vi "Grid_Init_v2.vi"(7 "resume":T1, 8 "Error in":errorcluster, 10 "Settings":T2={"Drift Correction Settings"={"Drift Correction every"=80, "Drift correction Pixels"=256, "Channel index (0-23)"=0, "MaxImagesBack"=2, "Threshold"=2, "Increment"=8, "max applied Drift Correction"=20, "Correct Drift"=TRUE, "Correlate"=0, "Correct z drift"=FALSE, "zdrift \nDuration (s)"=0.0}, "Spectroscopy Setting"={"Imaging Current"=1e-11, "ref Current"=7e-11, "tip Speed (m/s)"=2e-09, "Imaging Bias"=0.02, "ref Bias"=-0.1, "preSTS delay [ms]"=500, "STS z offset"=2e-10, "during Spec Bias (V)"=-0.1, "trigger1 < Hz"=0.0, "trigger 2 >Hz"=0.0, "autoStop"=FALSE, "Spectroscopy"=0, "PLL ON/OFF"=TRUE, "readjust setpoint every "=1, "z Reference"=FALSE, "Lock In"=TRUE}, "Misc"={"File name"="symmetric_node_zOff=200p", "Email when finished"="cornelius.krull@monash.edu,Dhaneesh.Gopalakrishnan@monash.edu,marina.castelli@monash.edu"}, "Grid Settings"={"type"=1, "type order"=1, "X pixel"=0, "Y pixel"=0, "Grid_Parms"={"center X (m)"=0.0, "center Y (m)"=0.0, "width (m)"=0.0, "height (m)"=0.0, "angle (deg)"=0.0}}} {"Grid Settings"."type order" items=["Line", "Grid"]; "Grid Settings"."type" items=["Line", "Grid"]; "Spectroscopy Setting"."Spectroscopy" items=["Bias", "zSpec"]; "Spectroscopy Setting"."trigger 2 >Hz" format="%#_6p"; "Spectroscopy Setting"."trigger1 < Hz" format="%#_6p"; "Spectroscopy Setting"."during Spec Bias (V)" format="%#_5p"; "Spectroscopy Setting"."STS z offset" format="%#_6p"; "Spectroscopy Setting"."ref Bias" format="%#_6p"; "Spectroscopy Setting"."Imaging Bias" format="%#_6p"; "Spectroscopy Setting"."tip Speed (m/s)" format="%.2p"; "Spectroscopy Setting"."ref Current" format="%#_6p"; "Spectroscopy Setting"."Imaging Current" format="%#_6p"; "Drift Correction Settings"."Correlate" items=["first Frame", "successive Frames"]; "Drift Correction Settings"."max applied Drift Correction" min=1 max=100 step=1 format="%.0p"; "Drift Correction Settings"."Threshold" min=1 step=1; "Drift Correction Settings"."Channel index (0-23)" items=["Current"=0, "Z (m)"=14]}, 11 "Application reference":refnum<vi>) -> (0 "error out":errorcluster, 1 "FileRefs":T3, 2 "Settings out":T2={"Drift Correction Settings"={"Drift Correction every"=80, "Drift correction Pixels"=256, "Channel index (0-23)"=0, "MaxImagesBack"=2, "Threshold"=2, "Increment"=8, "max applied Drift Correction"=20, "Correct Drift"=TRUE, "Correlate"=0, "Correct z drift"=FALSE, "zdrift \nDuration (s)"=0.0}, "Spectroscopy Setting"={"Imaging Current"=1e-11, "ref Current"=7e-11, "tip Speed (m/s)"=2e-09, "Imaging Bias"=0.02, "ref Bias"=-0.1, "preSTS delay [ms]"=500, "STS z offset"=2e-10, "during Spec Bias (V)"=-0.1, "trigger1 < Hz"=0.0, "trigger 2 >Hz"=0.0, "autoStop"=FALSE, "Spectroscopy"=0, "PLL ON/OFF"=TRUE, "readjust setpoint every "=1, "z Reference"=FALSE, "Lock In"=TRUE}, "Misc"={"File name"="symmetric_node_zOff=200p", "Email when finished"="cornelius.krull@monash.edu,Dhaneesh.Gopalakrishnan@monash.edu,marina.castelli@monash.edu"}, "Grid Settings"={"type"=1, "type order"=1, "X pixel"=0, "Y pixel"=0, "Grid_Parms"={"center X (m)"=0.0, "center Y (m)"=0.0, "width (m)"=0.0, "height (m)"=0.0, "angle (deg)"=0.0}}} caption="Settings" {"Grid Settings"."type order" items=["Line", "Grid"]; "Grid Settings"."type" items=["Line", "Grid"]; "Spectroscopy Setting"."Spectroscopy" items=["Bias", "zSpec"]; "Spectroscopy Setting"."trigger 2 >Hz" format="%#_6p"; "Spectroscopy Setting"."trigger1 < Hz" format="%#_6p"; "Spectroscopy Setting"."during Spec Bias (V)" format="%#_5p"; "Spectroscopy Setting"."STS z offset" format="%#_6p"; "Spectroscopy Setting"."ref Bias" format="%#_6p"; "Spectroscopy Setting"."Imaging Bias" format="%#_6p"; "Spectroscopy Setting"."tip Speed (m/s)" format="%.2p"; "Spectroscopy Setting"."ref Current" format="%#_6p"; "Spectroscopy Setting"."Imaging Current" format="%#_6p"; "Drift Correction Settings"."Correlate" items=["first Frame", "successive Frames"]; "Drift Correction Settings"."max applied Drift Correction" min=1 max=100 step=1 format="%.0p"; "Drift Correction Settings"."Threshold" min=1 step=1; "Drift Correction Settings"."Channel index (0-23)" items=["Current"=0, "Z (m)"=14]}, 3 "Application ref out":refnum<vi>, 5 "DC images":dbl[][][](array[numeric]))   [LabVIEW 2014]
uses:
  <userlib>/Nanonis Prog Interface V5/Nanonis Prog Interface.lvlib
panel:
  # "RUN smart tilt before starting the GRID\nImg Angle = 0  CHECK CUTOFF\nmove tip to reference point for tip height"
  # "z Spectroscopy"
  # "GRID points"
  # "Increase this if no Drift was detected for \na certain number of images"
  # "% of image size"
  # "RUN smart tilt before starting the GRID\nImg Angle = 0  CHECK CUTOFF\nmove tip to reference point for tip height"
  # "z Spectroscopy"
  # "GRID points"
  # "Increase this if no Drift was detected for \na certain number of images"
  # "% of image size"
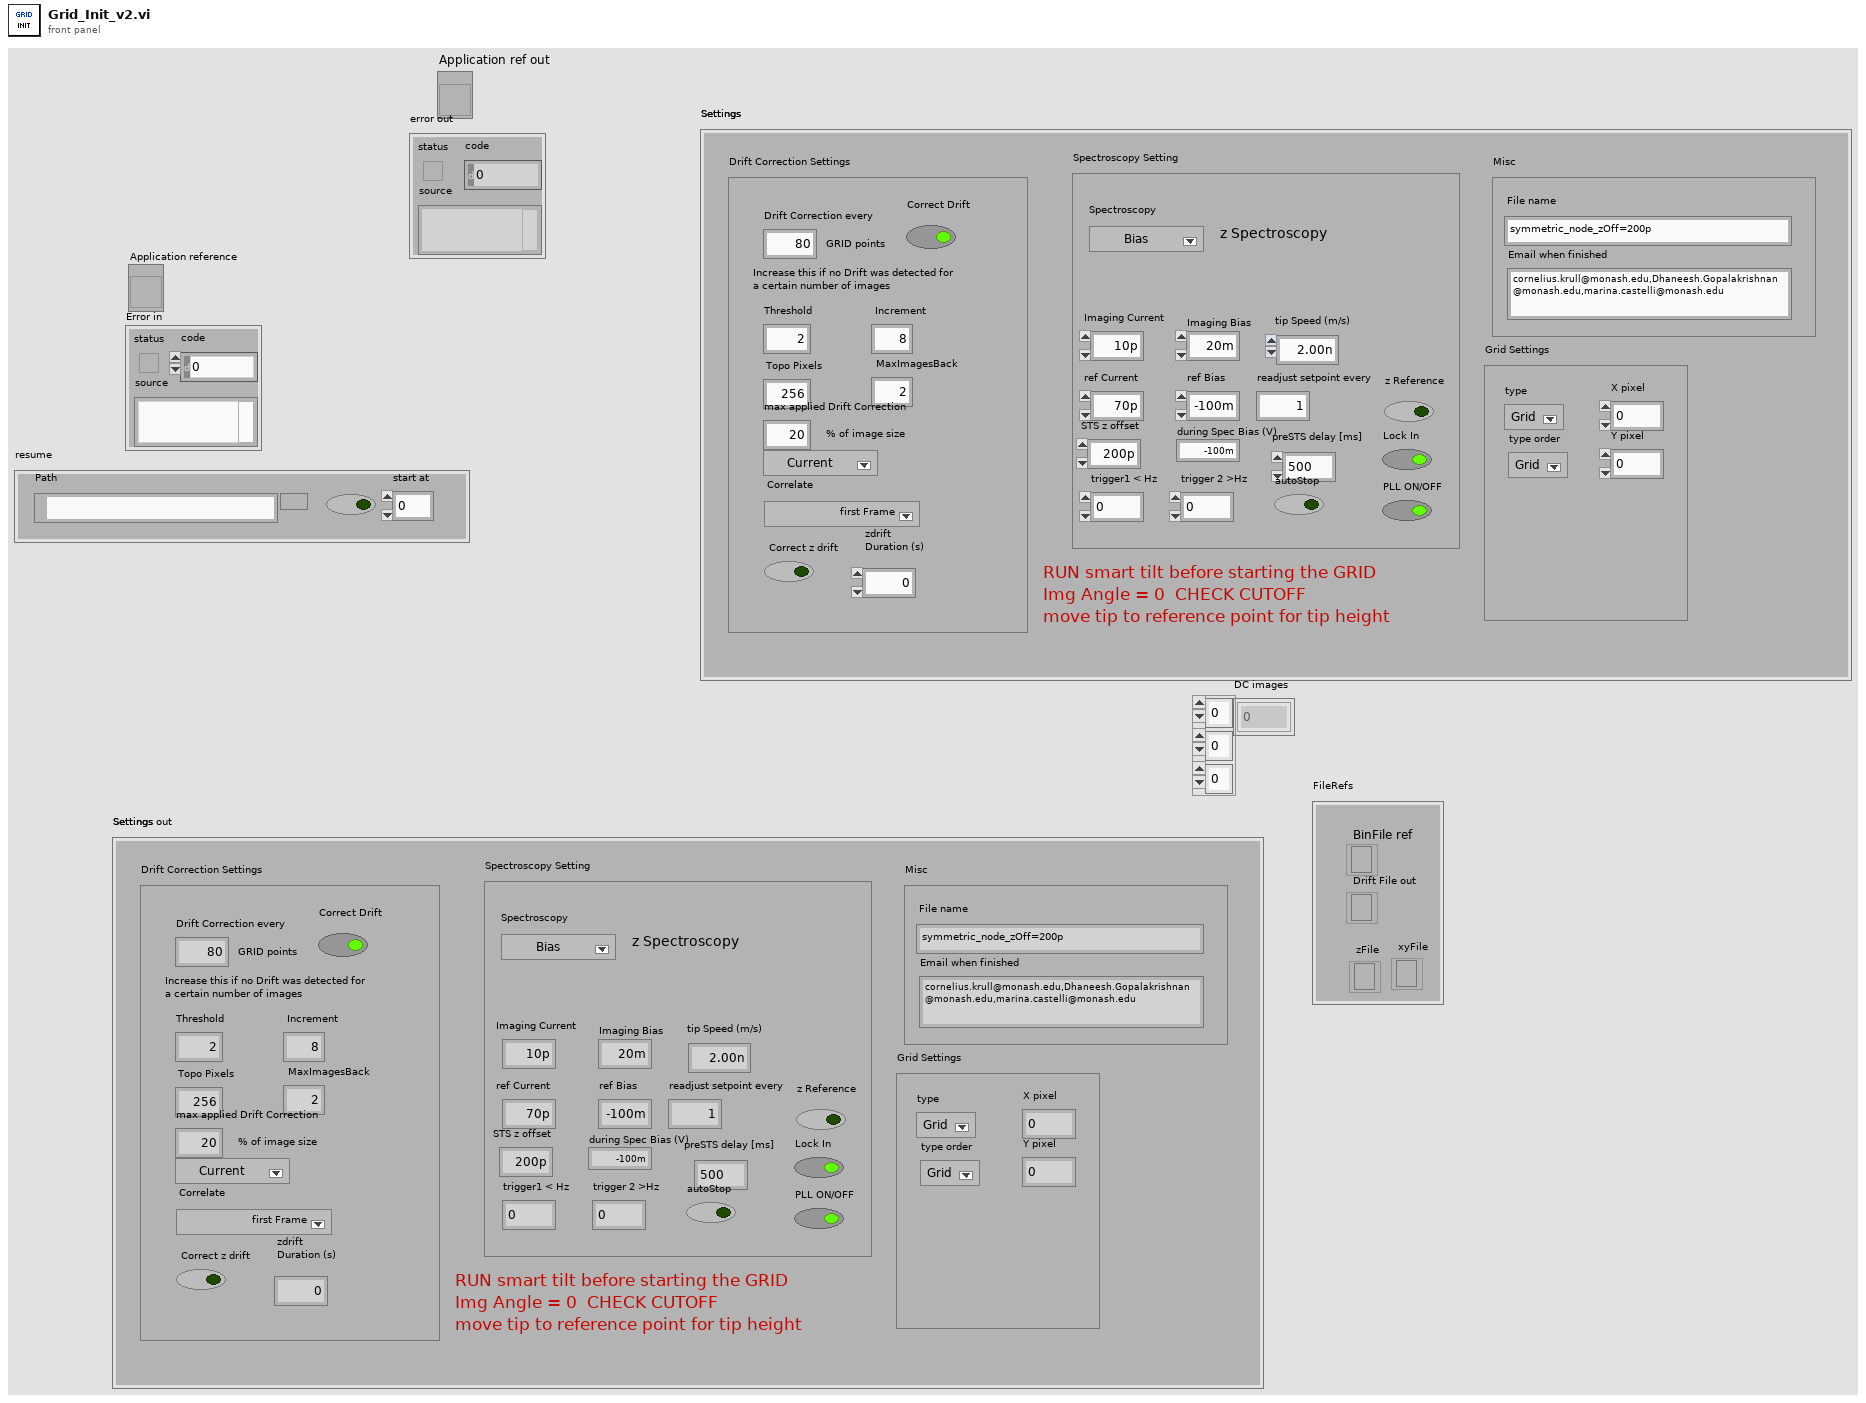
[diagram p1: front panel]
types:
  T1 = cluster{"resume Grid":bool, "Path":path, "start at":i32}
  T2 = cluster{"Drift Correction Settings":cluster{"Drift Correction every":i32, "Drift correction Pixels":i32, "Channel index (0-23)":u8, "MaxImagesBack":i32, "Threshold":i32, "Increment":i32, "max applied Drift Correction":i32, "Correct Drift":bool, "Correlate":u16, "Correct z drift":bool, "zdrift \nDuration (s)":dbl}, "Spectroscopy Setting":cluster{"Imaging Current":dbl, "ref Current":dbl, "tip Speed (m/s)":sgl, "Imaging Bias":dbl, "ref Bias":dbl, "preSTS delay [ms]":u32, "STS z offset":dbl, "during Spec Bias (V)":sgl, "trigger1 < Hz":sgl, "trigger 2 >Hz":sgl, "autoStop":bool, "Spectroscopy":u16, "PLL ON/OFF":bool, "readjust setpoint every ":i32, "z Reference":bool, "Lock In":bool}, "Misc":cluster{"File name":string, "Email when finished":string}, "Grid Settings":cluster{"type":u16, "type order":u16, "X pixel":i32, "Y pixel":i32, "Grid_Parms":cluster{"center X (m)":sgl, "center Y (m)":sgl, "width (m)":sgl, "height (m)":sgl, "angle (deg)":sgl}}}
  T3 = cluster{"Drift File out":refnum<file>, "zFile":refnum<file>, "BinFile ref":refnum<file>, "xyFile":refnum<file>}
  T4 = cluster{"type":u16, "type order":u16, "X pixel":i32, "Y pixel":i32, "Grid_Parms":cluster{"center X (m)":sgl, "center Y (m)":sgl, "width (m)":sgl, "height (m)":sgl, "angle (deg)":sgl}}
  T5 = cluster{"type":u16, "type order":u16, "X pixel":dbl, "Y pixel":dbl, "Grid_Parms":cluster{"center X (m)":sgl, "center Y (m)":sgl, "width (m)":sgl, "height (m)":sgl, "angle (deg)":sgl}}
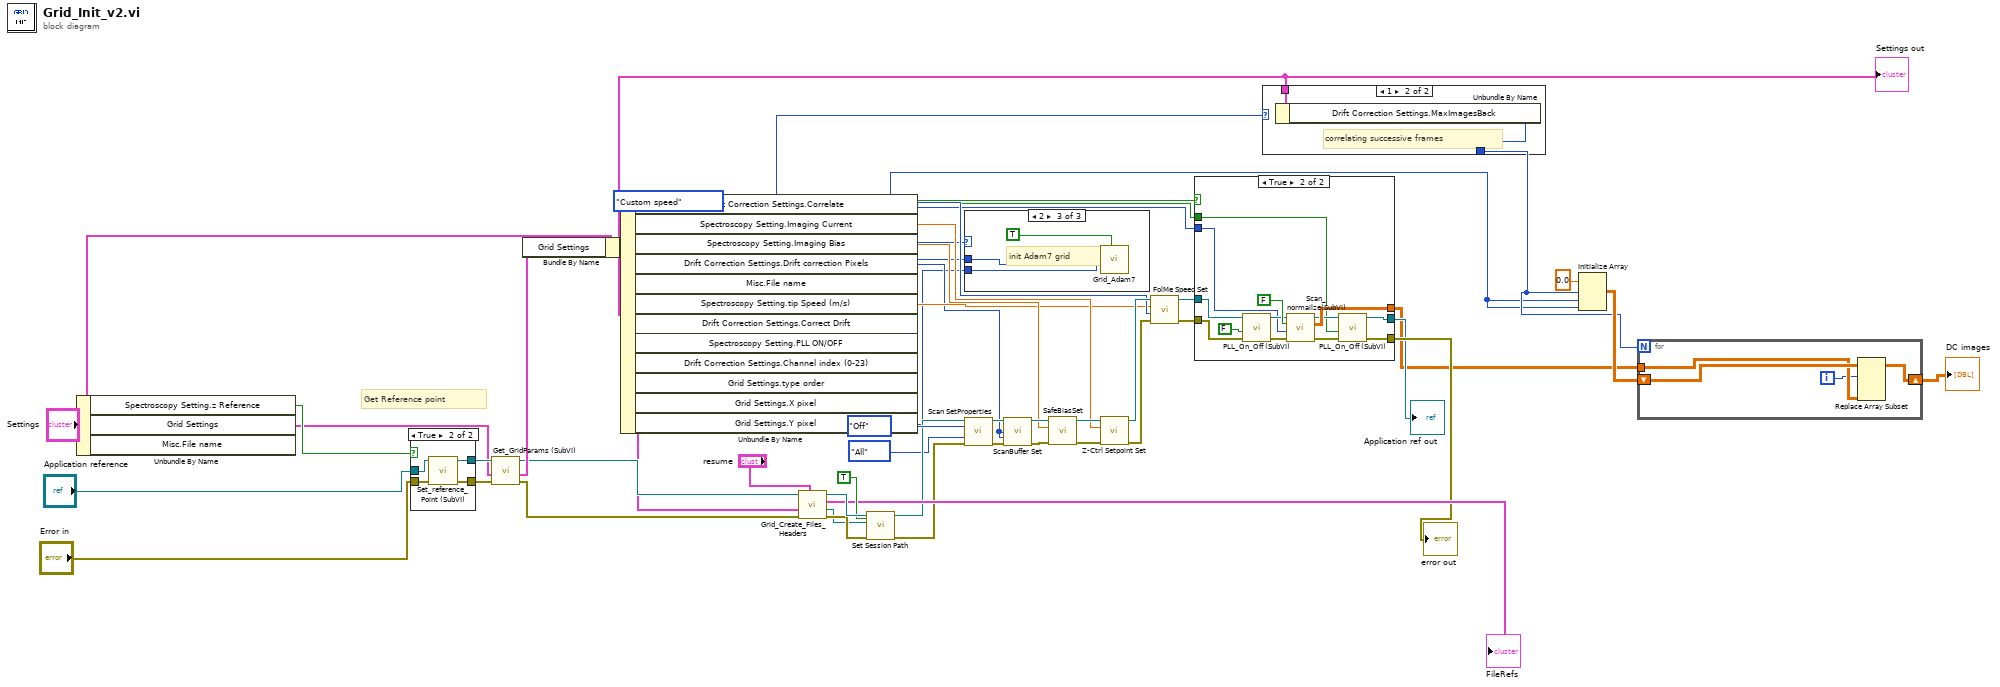
[diagram p0: block diagram]
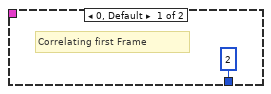
[diagram p4: hidden frame]
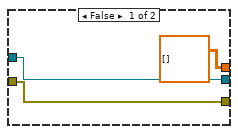
[diagram p5: hidden frame]
diagram:
  # "Get Reference point"
  n1 = Unbundle By Name("Settings") -> ("Spectroscopy Setting.z Reference"=w48:bool, "Grid Settings"=w45:T4)  [unwired: 1 out]
  n2 = case shown="True" w48 {
    tunnel: "Application reference" -> [w52 w56]
    tunnel: "Error in" -> [w51 w55]
    tunnel: [w52 w54] -> w47
    tunnel: [w51 w53] -> w46
    frame False {
    }
    frame True {
      n3 = call "Set_reference_Point (SubVI).vi"("error in (no error)"=w55, "Application in"=w56) -> ("error out"=w53:errorcluster, "Application out"=w54:refnum<vi>)  [unwired: 8 in]
    }
  }
  n4 = call "Get_GridParams (SubVI).vi"("error in (no error)"=w46, "Grid Settings"=w45, "Application in"=w47) -> ("error out"=w41:errorcluster, "Grid Settings"=w43:T5, "Application out"=w42:refnum<vi>)  [unwired: 5 in, 1 out]
  n5 = Bundle By Name(cluster="Settings", "Grid Settings"=w43) -> (w5:T2)
  "Settings out" <- w5
  n6 = Unbundle By Name(w5) -> ("Drift Correction Settings.Correlate"=w6:u16, "Spectroscopy Setting.Imaging Current"=w25:dbl, "Spectroscopy Setting.Imaging Bias"=w28:dbl, "Drift Correction Settings.Drift correction Pixels"=w7:i32, "Spectroscopy Setting.tip Speed (m/s)"=w21:sgl, "Drift Correction Settings.Correct Drift"=w16:bool, "Spectroscopy Setting.PLL ON/OFF"=w15:bool, "Drift Correction Settings.Channel index (0-23)"=w14:u8, "Grid Settings.type order"=w4:u16, "Grid Settings.X pixel"=w3:i32, "Grid Settings.Y pixel"=w2:i32)  [unwired: 1 out]
  n7 = call "Grid_Create_Files_Headers.vi"("resume"="resume", "Error in (no error)"=w41, "Settings"=w5, "Application ref in"=w42) -> ("error out"=w38:errorcluster, "topoFilePath"=w13:path, "FileRefs"=→"FileRefs":T3, "Application ref out"=w40:refnum<vi>)  [unwired: 4 in]
  n8 = call <userlib>:"Set Session Path.vi"("Save settings to previous? (False)"=TRUE, "error in (no error)"=w38, "Session Folder"=w13, "Application ref in"=w40) -> ("error out"=w32:errorcluster, "Application ref out"=w33:refnum<vi>)  [unwired: 6 in]
  n9 = case shown="2" w4 {
    tunnel: w3 -> [_ _ w58]
    tunnel: w2 -> [_ _ w57]
    frame 0, Default {
    }
    frame 1 {
    }
    frame 2 {
      # "init Adam7 grid"
      n10 = call "Grid_Adam7.vi"("reset"=TRUE, "py 2"=w57, "px 2"=w58) -> ()  [unwired: 7 in, 2 out]
    }
  }
  n11 = call <userlib>:"Scan SetProperties.vi"("Application ref in"=w33, "Continuous scan"=enum16{"No change", "On", "Off"}."Off", "Auto save"=enum16{"No change", "All", "Next", "Off"}."All", "Error in (no error)"=w32) -> ("Application ref out"=w35:refnum<vi>, "Error out"=w34:errorcluster)  [unwired: 10 in]
  n12 = call <userlib>:"ScanBuffer Set.vi"("Application ref in"=w35, "Pixels"=w7, "Lines"=w7, "error in (no error)"=w34) -> ("Application ref out"=w30:refnum<vi>, "error out"=w29:errorcluster)  [unwired: 10 in]
  n13 = call "SafeBiasSet.vi"("Application ref in"=w30, "Bias (V)"=w28, "error in (no error)"=w29) -> ("Application ref out"=w26:refnum<vi>, "Error out"=w27:errorcluster)  [unwired: 6 in]
  n14 = call <userlib>:"Z-Ctrl Setpoint Set.vi"("error in (no error)"=w27, "Z Controller setpoint"=w25, "Application ref in"=w26) -> ("error out"=w23:errorcluster, "Application ref out"=w24:refnum<vi>)  [unwired: 7 in]
  n15 = call <userlib>:"FolMe Speed Set.vi"("error in (no error)"=w23, "Speed Setting (Custom)"=enum32{"Scan speed", "Custom speed"}."Custom speed", "Speed (m/s)"=w21, "Application ref in"=w24) -> ("error out"=w19:errorcluster, "Application ref out"=w20:refnum<vi>)  [unwired: 4 in]
  n16 = case shown="True" w16 {
    tunnel: [dbl[][] [] ("Array") w75] -> w10
    tunnel: w20 -> [w62 w73]
    tunnel: [w62 w69] -> w17
    tunnel: w19 -> [w60 w68]
    tunnel: [w60 w65] -> w18
    tunnel: w15 -> [_ w64]
    tunnel: w14 -> [_ w63]
    frame False {
    }
    frame True {
      n17 = call "PLL_On_Off (SubVI).vi"("error in (no error)"=w68, "Output ON/OFF (F=OFF)"=FALSE, "Application in"=w73) -> ("error out"=w67:errorcluster, "Application out"=w72:refnum<vi>)  [unwired: 7 in]
      n18 = call "Scan_normailze(SubVI).vi"("error in (no error)"=w67, "Channel index (0-23)"=w63, "Normalization"=FALSE ("Boolean"), "Application in"=w72) -> ("error out"=w66:errorcluster, "Array"=w75:dbl[][], "Application out"=w70:refnum<vi>)  [unwired: 5 in]
      n19 = call "PLL_On_Off (SubVI).vi"("error in (no error)"=w66, "Output ON/OFF (F=OFF)"=w64, "Application in"=w70) -> ("error out"=w65:errorcluster, "Application out"=w69:refnum<vi>)  [unwired: 7 in]
    }
  }
  "Application ref out" <- w17
  "error out" <- w18
  n20 = case shown="1" w6 {
    tunnel: w5 -> [_ w78]
    tunnel: [2 ("MaxImagesBack") w77] -> w9
    frame 0, Default {
      # "Correlating first Frame"
    }
    frame 1 {
      # "correlating successive frames"
      n21 = Unbundle By Name(w78) -> ("Drift Correction Settings.MaxImagesBack"=w77:i32)
    }
  }
  n22 = Initialize Array(0.0 ("element"), w9, w7, w7) -> (w11:dbl[][][])
  n23 = for {
    N: w9 -> [_]
    tunnel: w10 -> [w81]
    shift-right: [w80] -> w8
    shift-left: w11 -> [w82]
    i -> [w79]
    n24 = Replace Array Subset(array=w82, new element=w81, index (dim 0)=w79) -> (w80:dbl[][][])  [unwired: 2 in]
  }
  "DC images" <- w8
